vi "Step_Complete.vi"(8 "error in":errorcluster, 11 "System data in":T1) -> (0 "error out":errorcluster, 1 "Car Position":variant, 2 "State":T3, 3 "System data out":T1)   [LabVIEW 2023]
uses:
  Controls/State.ctl
  Controls/System_Data.ctl
  Controls/Wash Options.ctl
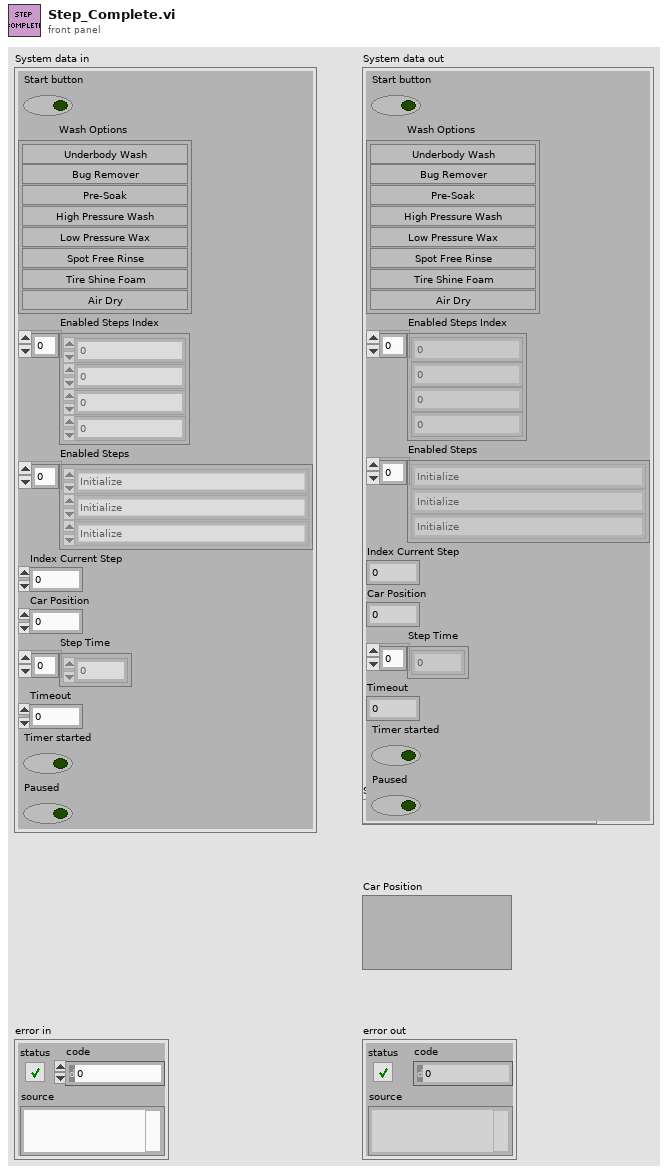
[diagram p1: front panel]
types:
  T1 = typedef "System_Data.ctl" = cluster{"Start button":bool, "Wash Options":T2, "Enabled Steps Index":i32[], "Enabled Steps ":T3[], "Index Current Step":i32, "Car Position":u8, "Step Time":dbl[], "Timeout":i32, "Timer started":bool, "Paused":bool}
  T2 = typedef "Wash Options.ctl" = cluster{"Underbody Wash":bool, "Bug Remover":bool, "Pre-Soak":bool, "High Pressure Wash":bool, "Low Pressure Wax":bool, "Spot Free Rinse":bool, "Tire Shine Foam":bool, "Air Dry":bool}
  T3 = typedef "State.ctl" = enum16{"Initialize", "Wait for Something", "Step Completed", "Save Wash Options", "Start Process", "Car Position", "Order Steps to follow", "Underbody Wash", "Bug Remover", "Pre-Soak", "High Pressure Wash", "Low Pressure Wax", "Spot Free Rinse", "Tire Shine Foam", "Air Dry", "Vehicle out of position", "Exit", "Process Complete", "Stop Application"}
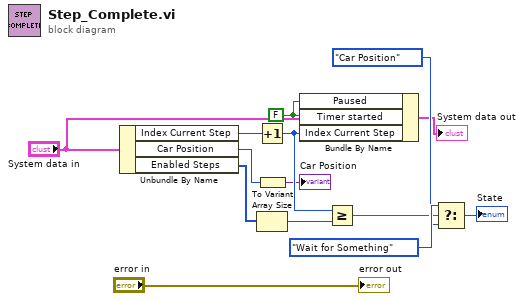
[diagram p0: block diagram]
diagram:
  w1 = FALSE
  n1 = Unbundle By Name("System data in") -> ("Index Current Step"=w4:i32, "Car Position"=w6:u8, "Enabled Steps"=w9:T3[])
  n2 = Increment(x=w4) -> (x+1=w8:i32)
  n3 = Array Size(array=w9) -> (size(s)=w10:i32)
  n4 = To Variant(anything=w6) -> (Variant=→"Car Position":variant)
  n5 = Bundle By Name(cluster="System data in", "Paused"=w1, "Timer started"=w1, "Index Current Step"=w8) -> (→"System data out":T1)
  n6 = Greater Or Equal?(x=w8, y=w10) -> (x >= y?=w11:bool)
  n7 = Select(t=State."Wait for Something" ("State"), s=w11, f=State."Car Position" ("State")) -> (s? t:f=→"State":T3)
  "error out" <- "error in"
